vi "Signal Generation.vi"(5 "Sampling info":cluster{"Fs":dbl, "#s":dbl}, 7 "error in (no error)":errorcluster, 8 "Queue in":refnum<queue>) -> (0 "error out":errorcluster)   [LabVIEW 2019]
uses:
  Type Definitions/Machine States/Oscillator State.ctl
  Type Definitions/DataInOut.ctl
  <vilib>/Waveform/WDTOps.llb/WDT Waveform Duration DBL.vi
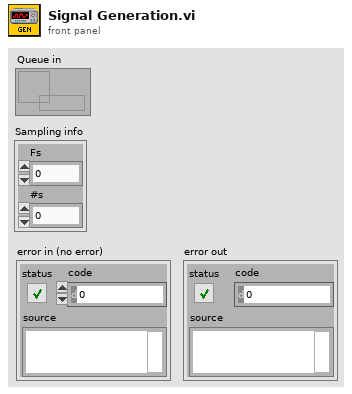
[diagram p1: front panel]
types:
  T1 = typedef "Oscillator State.ctl" = enum16{"Idle", "Attack", "Decay", "Sustain", "Release"}
  T2 = typedef "DataInOut.ctl" = enum16{"Write", "Read"}
  T3 = typedef "UI.ctl" = cluster{"Play sound":bool, "Stop Application":bool, "Oscillator":T4, "VCA":T6, "Lowpass filter":T7, "Tremolo":T8}
  T4 = typedef "UIOscillatorParam.ctl" = cluster{"Waveform Type":enum16{"Sine Wave", "Triangle Wave", "Square Wave", "Sawtooth Wave"}, "Frequency":dbl, "Pulse Width":dbl, "Sub oscillator":T5}
  T5 = typedef "Sub Oscillalator Type.ctl" = enum16{"Off", "One Octave", "Two Octaves"}
  T6 = typedef "UIADSRParam.ctl" = cluster{"Volume":dbl, "A":i8, "S":i8, "R":i8, "D":i8}
  T7 = typedef "UILowpassParam.ctl" = cluster{"On / Off":bool, "Cutoff":dbl}
  T8 = typedef "UITremolo.ctl" = cluster{"On / Off":bool, "Frequency":dbl, "Rate":dbl}
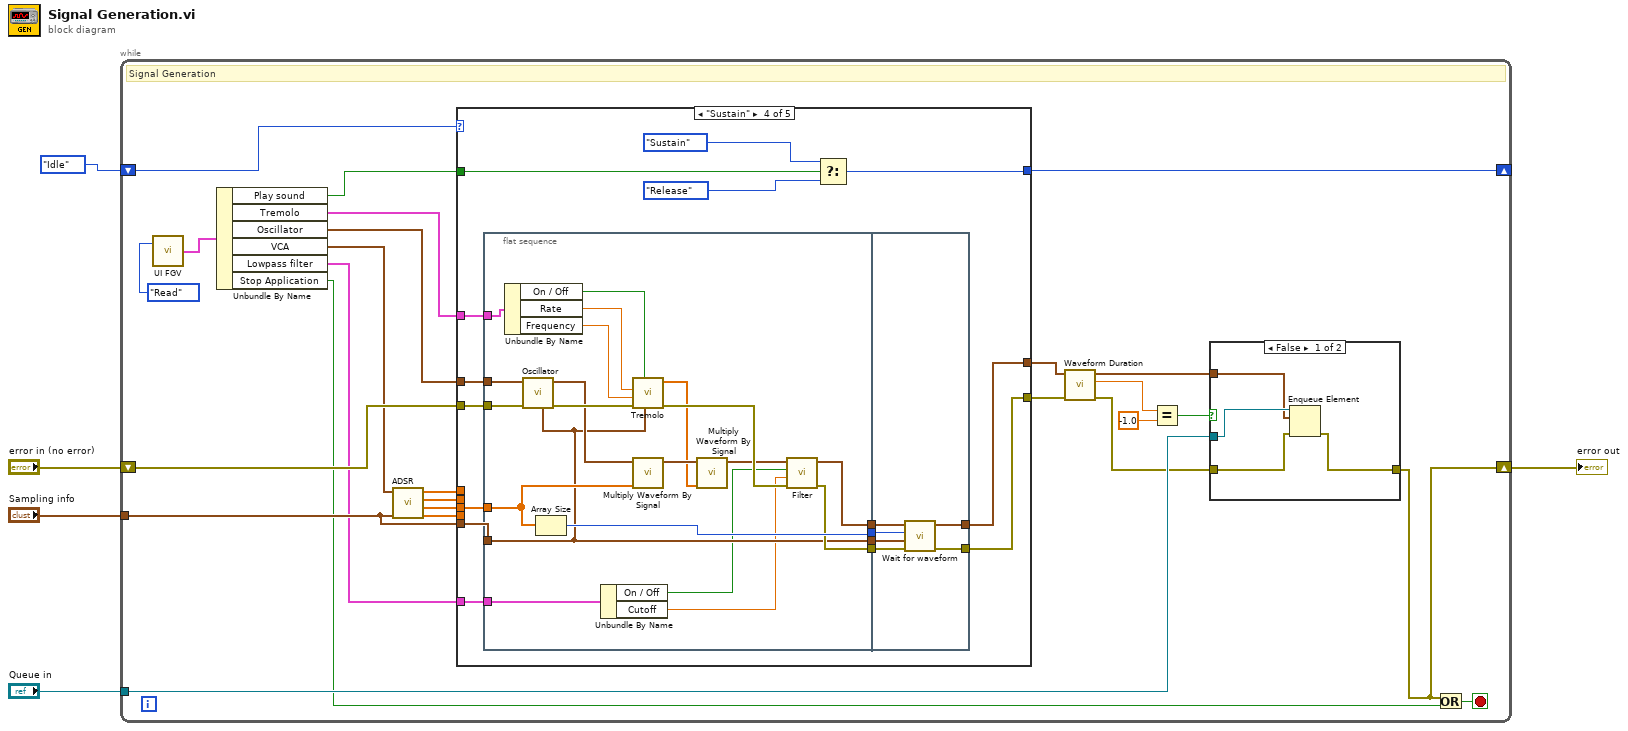
[diagram p0: block diagram]
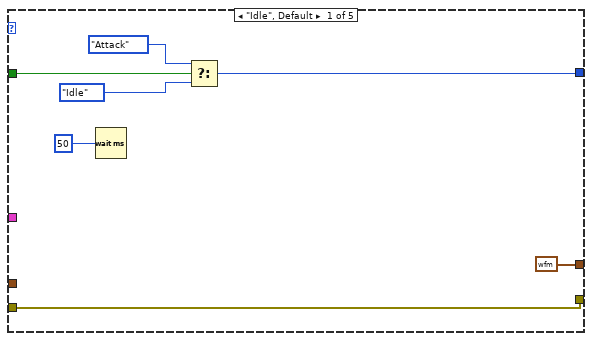
[diagram p3: hidden frame]
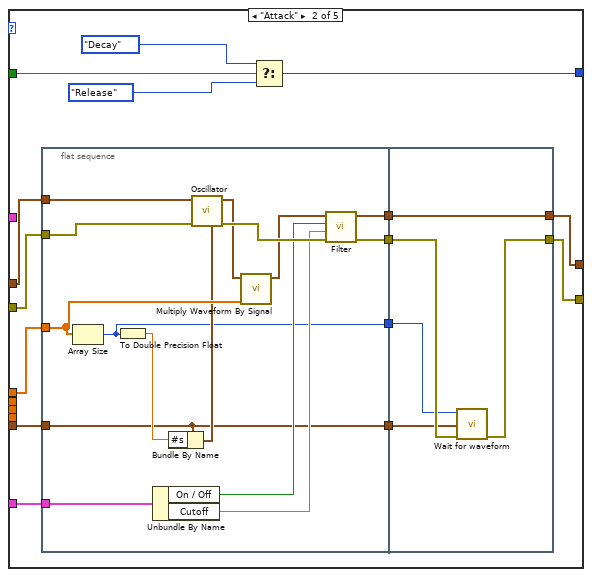
[diagram p4: hidden frame]
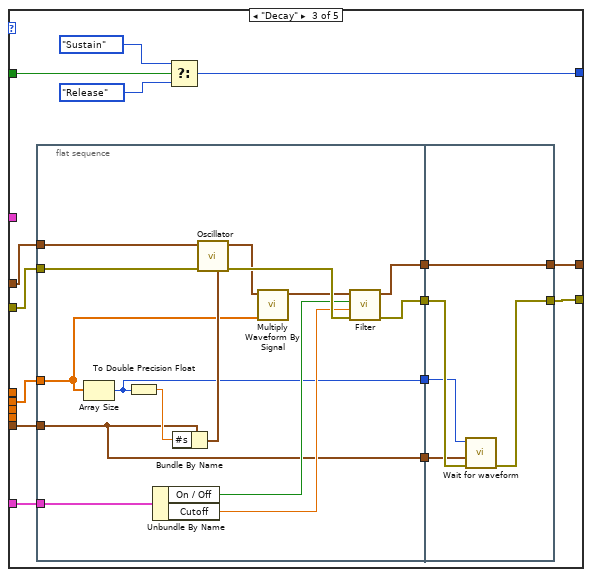
[diagram p5: hidden frame]
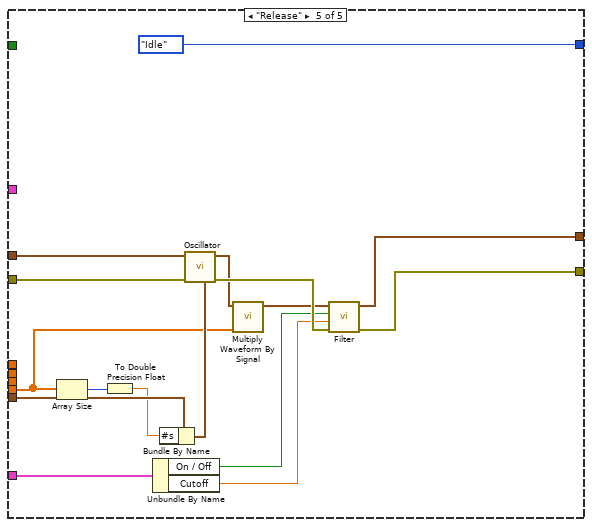
[diagram p6: hidden frame]
diagram:
  n1 = while {
    shift-right: [w29] -> _
    shift-left: Oscillator_State."Idle" -> [w31]
    tunnel: "Sampling info" -> [w18]
    shift-right: [w19] -> w4
    shift-left: "error in (no error)" -> [w30]
    tunnel: "Queue in" -> [w22]
    stop <- w28 stop-if-true
    # "Signal Generation"
    n2 = call "UI FGV.vi"("Mode"=DataInOut."Read" ("Enum")) -> ("Data out"=w16:T3)  [unwired: 1 in]
    n3 = Unbundle By Name(w16) -> ("Play sound"=w15:bool, "Tremolo"=w11:T8, "Oscillator"=w12:T4, "VCA"=w13:T6, "Lowpass filter"=w10:T7, "Stop Application"=w14:bool)
    n4 = call "ADSR.vi"("Sampling info"=w18, "ADSR Params"=w13) -> ("R"=w9:dbl[], "S"=w8:dbl[], "D"=w7:dbl[], "A"=w6:dbl[])  [unwired: 6 in]
    n5 = case shown="\"Sustain\"" w31 {
      tunnel: [w41 w57 w91 w127 Oscillator_State."Idle"] -> w29
      tunnel: w30 -> [w38 w52 w86 w123 w159]
      tunnel: w18 -> [_ w53 w87 w124 w170]
      tunnel: [w38 w44 w89 w125 w164] -> w26
      tunnel: [waveform(dbl) {"t0"=timestamp(0 s since 1904-01-01), "dt"=1.0, "Y"=[]} ("signal out") w55 w90 w126 w165] -> w27
      tunnel: w6 -> [_ w54 _ _ _]
      tunnel: w7 -> [_ _ w88 _ _]
      tunnel: w8 -> [_ _ _ w114 _]
      tunnel: w9 -> [_ _ _ _ w160]
      tunnel: w15 -> [w37 w47 w81 w119 _]
      tunnel: w12 -> [_ w46 w80 w118 w158]
      tunnel: w11 -> [_ _ _ w117 _]
      tunnel: w10 -> [_ w45 w79 w115 w157]
      frame "Idle", Default {
        n6 = Wait (ms)(milliseconds to wait=u32 50) -> ()  [unwired: 1 out]
        n7 = Select(t=Oscillator_State."Attack", s=w37, f=Oscillator_State."Idle") -> (s? t:f=w41:T1)
      }
      frame "Attack" {
        n8 = flat-sequence {
          tunnel: w54 -> [w68]
          tunnel: w53 -> [w62]
          tunnel: w52 -> [w66]
          tunnel: [w72] -> w51
          tunnel: [w71] -> w50
          tunnel: [w62] -> w49
          tunnel: [w61] -> w48
          tunnel: w46 -> [w60]
          tunnel: w45 -> [w59]
          tunnel: [w76] -> w44
          tunnel: [w78] -> w55
          tunnel: w51 -> [w78]
          tunnel: w50 -> [w77]
          tunnel: w49 -> [w75]
          tunnel: w48 -> [w74]
          frame #0 {
            n9 = Array Size(array=w68) -> (size(s)=w61:i32)
            n10 = To Double Precision Float(number=w61) -> (double precision float=w73:dbl)
            n11 = Unbundle By Name(w59) -> ("On / Off"=w64:bool, "Cutoff"=w65:dbl)
            n12 = Bundle By Name(cluster=w62, "#s"=w73) -> (w63:cluster{"Fs":dbl, "#s":dbl})
            n13 = call "Oscillator.vi"("Sampling info"=w63, "Error in"=w66, "Parameters"=w60) -> ("Error out"=w70:errorcluster, "Waveform out"=w67:waveform(dbl))  [unwired: 7 in]
            n14 = call "Multiply Waveform By Signal.vi"("Signal in"=w68, "Waveform in"=w67) -> ("Waveform out"=w69:waveform(dbl))  [unwired: 5 in]
            n15 = call "Filter.vi"("error in"=w70, "Cutoff freq (Hz)"=w65, "On / Off"=w64, "signal in"=w69) -> ("error out"=w71:errorcluster, "signal out"=w72:waveform(dbl))  [unwired: 2 in]
          }
          frame #1 {
            n16 = call "Wait for waveform.vi"("Error in"=w77, "Sampling info"=w75, "Samples"=w74) -> ("Error out"=w76:errorcluster)  [unwired: 8 in]
          }
        }
        n17 = Select(t=Oscillator_State."Decay", s=w47, f=Oscillator_State."Release") -> (s? t:f=w57:T1)
      }
      frame "Decay" {
        n18 = flat-sequence {
          tunnel: w88 -> [w101]
          tunnel: w87 -> [w96]
          tunnel: w86 -> [w100]
          tunnel: [w106] -> w85
          tunnel: [w105] -> w84
          tunnel: [w97] -> w83
          tunnel: [w96] -> w82
          tunnel: w80 -> [w95]
          tunnel: w79 -> [w94]
          tunnel: [w111] -> w89
          tunnel: [w113] -> w90
          tunnel: w85 -> [w113]
          tunnel: w84 -> [w112]
          tunnel: w83 -> [w110]
          tunnel: w82 -> [w109]
          frame #0 {
            n19 = Array Size(array=w101) -> (size(s)=w97:i32)
            n20 = To Double Precision Float(number=w97) -> (double precision float=w108:dbl)
            n21 = Unbundle By Name(w94) -> ("On / Off"=w99:bool, "Cutoff"=w98:dbl)
            n22 = Bundle By Name(cluster=w96, "#s"=w108) -> (w107:cluster{"Fs":dbl, "#s":dbl})
            n23 = call "Oscillator.vi"("Sampling info"=w107, "Error in"=w100, "Parameters"=w95) -> ("Error out"=w104:errorcluster, "Waveform out"=w103:waveform(dbl))  [unwired: 7 in]
            n24 = call "Multiply Waveform By Signal.vi"("Signal in"=w101, "Waveform in"=w103) -> ("Waveform out"=w102:waveform(dbl))  [unwired: 5 in]
            n25 = call "Filter.vi"("error in"=w104, "Cutoff freq (Hz)"=w98, "On / Off"=w99, "signal in"=w102) -> ("error out"=w105:errorcluster, "signal out"=w106:waveform(dbl))  [unwired: 2 in]
          }
          frame #1 {
            n26 = call "Wait for waveform.vi"("Error in"=w112, "Sampling info"=w109, "Samples"=w110) -> ("Error out"=w111:errorcluster)  [unwired: 8 in]
          }
        }
        n27 = Select(t=Oscillator_State."Sustain", s=w81, f=Oscillator_State."Release") -> (s? t:f=w91:T1)
      }
      frame "Sustain" {
        n28 = flat-sequence {
          tunnel: w114 -> [w145]
          tunnel: w124 -> [w134]
          tunnel: w123 -> [w142]
          tunnel: [w147] -> w122
          tunnel: [w134] -> w121
          tunnel: [w141] -> w120
          tunnel: w118 -> [w140]
          tunnel: w117 -> [w139]
          tunnel: [w135] -> w116
          tunnel: w115 -> [w130]
          tunnel: [w153] -> w125
          tunnel: [w154] -> w126
          tunnel: w122 -> [w154]
          tunnel: w121 -> [w152]
          tunnel: w120 -> [w151]
          tunnel: w116 -> [w150]
          frame #0 {
            n29 = Unbundle By Name(w139) -> ("On / Off"=w136:bool, "Rate"=w137:dbl, "Frequency"=w138:dbl)
            n30 = call "Oscillator.vi"("Sampling info"=w134, "Error in"=w142, "Parameters"=w140) -> ("Error out"=w149:errorcluster, "Waveform out"=w146:waveform(dbl))  [unwired: 7 in]
            n31 = Array Size(array=w145) -> (size(s)=w141:i32)
            n32 = Unbundle By Name(w130) -> ("On / Off"=w132:bool, "Cutoff"=w131:dbl)
            n33 = call "Tremolo.vi"("Sampling info"=w134, "On / Off"=w136, "error in"=w149, "Freq"=w138, "Rate"=w137) -> ("error out"=w148:errorcluster, "signal out"=w133:dbl[])  [unwired: 3 in]
            n34 = call "Multiply Waveform By Signal.vi"("Signal in"=w145, "Waveform in"=w146) -> ("Waveform out"=w144:waveform(dbl))  [unwired: 5 in]
            n35 = call "Multiply Waveform By Signal.vi"("Signal in"=w133, "Waveform in"=w144) -> ("Waveform out"=w143:waveform(dbl))  [unwired: 5 in]
            n36 = call "Filter.vi"("error in"=w148, "Cutoff freq (Hz)"=w131, "On / Off"=w132, "signal in"=w143) -> ("error out"=w135:errorcluster, "signal out"=w147:waveform(dbl))  [unwired: 2 in]
          }
          frame #1 {
            n37 = call "Wait for waveform.vi"("Error in"=w150, "Sampling info"=w152, "Samples"=w151) -> ("Error out"=w153:errorcluster)  [unwired: 8 in]
          }
        }
        n38 = Select(t=Oscillator_State."Sustain", s=w119, f=Oscillator_State."Release") -> (s? t:f=w127:T1)
      }
      frame "Release" {
        n39 = Array Size(array=w160) -> (size(s)=w169:i32)
        n40 = To Double Precision Float(number=w169) -> (double precision float=w168:dbl)
        n41 = Unbundle By Name(w157) -> ("On / Off"=w155:bool, "Cutoff"=w156:dbl)
        n42 = Bundle By Name(cluster=w170, "#s"=w168) -> (w167:cluster{"Fs":dbl, "#s":dbl})
        n43 = call "Oscillator.vi"("Sampling info"=w167, "Error in"=w159, "Parameters"=w158) -> ("Error out"=w163:errorcluster, "Waveform out"=w161:waveform(dbl))  [unwired: 7 in]
        n44 = call "Multiply Waveform By Signal.vi"("Signal in"=w160, "Waveform in"=w161) -> ("Waveform out"=w162:waveform(dbl))  [unwired: 5 in]
        n45 = call "Filter.vi"("error in"=w163, "Cutoff freq (Hz)"=w156, "On / Off"=w155, "signal in"=w162) -> ("error out"=w164:errorcluster, "signal out"=w165:waveform(dbl))  [unwired: 2 in]
      }
    }
    n46 = call-poly <vilib>:"Waveform Duration.vi"("error in (no error)"=w26, "waveform in"=w27) -> ("error out"=w21:errorcluster, "duration"=w25:dbl, "waveform out"=w20:waveform(dbl))  [unwired: 7 in]
    n47 = Equal?(x=w25, y=-1.0) -> (x = y?=w23:bool)
    n48 = case shown="False" w23 {
      tunnel: w22 -> [w35 _]
      tunnel: w21 -> [w34 w36]
      tunnel: [w33 w36] -> w19
      tunnel: w20 -> [w32 _]
      frame False {
        n49 = Enqueue Element(queue=w35, element=w32, error in (no error)=w34) -> (error out=w33:errorcluster)  [unwired: 1 in, 2 out]
      }
      frame True {
      }
    }
    n50 = Or(x=w19, y=w14) -> (x .or. y?=w28:bool)
  }
  "error out" <- w4
